vi "Get Data_old.vi"(7 "error in":errorcluster, 10 "Alicat Device in":refnum<class "Alicat Device.lvclass">) -> (0 "error out":errorcluster, 2 "Base Data Lib:Data":refnum<class "Data.lvclass">, 3 "Alicat Device out":refnum<class "Alicat Device.lvclass">)   [LabVIEW 2014, in "Alicat Device.lvclass"]
doc: "Retrieve the data from the Alicat device. The Alicat device takes the address and returns data in a string format in the string <b>DataOut</b>. The data returned is also repackaged into the object <b>Alicat Data</b>."
uses:
  Alicat Device.lvclass
  Reusable/Data/Data.lvclass
  Alicat Device.lvclass/Alicat Device.ctl
  Data/Alicat Data.lvclass
  Reusable/Session APIs/Serial/Public/Get Data/Get String.vi
  Reusable/Session APIs/Text Communication/Text Device Session.lvclass
panel:
  out "DataOut":string
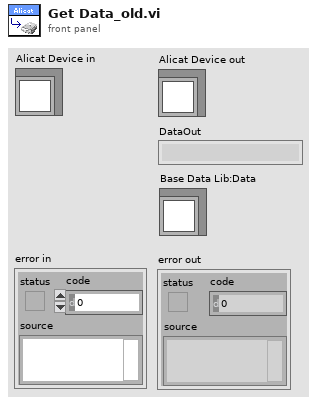
[diagram p1: front panel]
types:
  T1 = typedef "Session - Root.lvclass/Session Handle.ctl" = refnum<data-value>
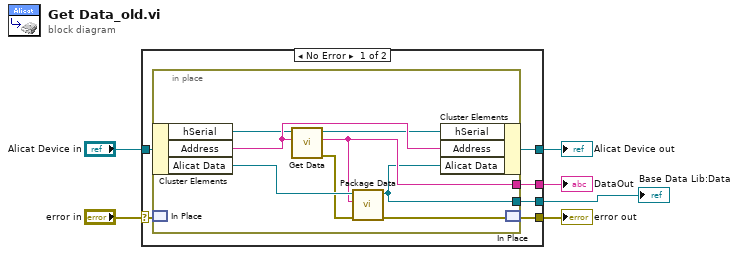
[diagram p0: block diagram]
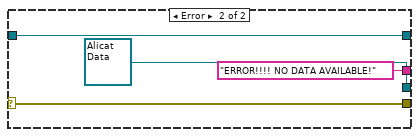
[diagram p2: hidden frame]
diagram:
  n1 = case shown="No Error" "error in" {
    selector: "error in" -> [w11 w24]
    tunnel: "Alicat Device in" -> [w12 w23]
    tunnel: [w9 w24] -> w2
    tunnel: [w10 w23] -> w5
    tunnel: [w8 "ERROR!!!! NO DATA AVAILABLE!" ("DataOut")] -> w4
    tunnel: [w7 refnum<class "Alicat Data.lvclass"> refnum ("Alicat Data out")] -> w1
    frame No Error {
      n2 = in-place {
        in-place-border: [w16] -> w8
        in-place-border: [w15] -> w7
        n3 = in-place-cluster #1(w12) -> ("hSerial"=w14:T1, "Address"=w19:string, "Alicat Data"=w20:refnum<class "Alicat Data.lvclass">)
        n4 = in-place-match #2(w11) -> ()  [unwired: 1 out]
        n5 = call-poly "Get Data.vi"("CMD"=w19, "handle in"=w14) -> ("error out"=w18:errorcluster, "DataOut"=w16:string, "handle out"=w13:T1)  [unwired: 7 in]
        n6 = call-dynamic "Package Data.vi"("error in"=w18, "DataIn"=w16, "Alicat Data in"=w20) -> ("error out"=w17:errorcluster, "Alicat Data out"=w15:refnum<class "Alicat Data.lvclass">)  [unwired: 7 in]
        n7 = in-place-cluster #1("hSerial"=w13, "Address"=w19, "Alicat Data"=w15) -> (w10:refnum<class "Alicat Device.lvclass">)
        n8 = in-place-match #2(w17) -> (w9:errorcluster)
      }
    }
    frame Error {
    }
  }
  "error out" <- w2
  "Alicat Device out" <- w5
  "DataOut" <- w4
  "Base Data Lib:Data" <- w1
